vi "Set Output Operation State.vi"(0 "VISA resource name":refnum<visa-resource-name>, 1 "Voltage Setpoint (0 V)":dbl format="%#.6g", 2 "Current Setpoint (0 A)":dbl format="%#.6g", 5 "Mode (0: Off)":i32(ring) items=["Off", "Standby", "Charge", "Discharge", "Battery"], 7 "Enable":T1, 11 "error in (no error)":errorcluster, 12 "Power Setpoint (0 W)":dbl format="%#.6g", 13 "Resistance Setpoint (0 Ohms)":dbl format="%#.6g") -> (4 "VISA resource name out":refnum<visa-resource-name>, 15 "error out":errorcluster)   [LabVIEW 2020, in "NH Research Regenerative Test Series.lvlib"]
doc: "This command sets the operation mode and settings."
uses:
  Drivers-Essentials/NH Research Regenerative Test Series.lvlib
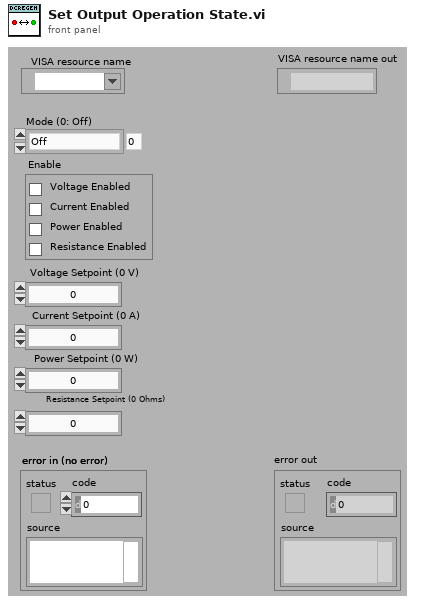
[diagram p1: front panel]
types:
  T1 = cluster{"Voltage Enabled":bool, "Current Enabled":bool, "Power Enabled":bool, "Resistance Enabled":bool}
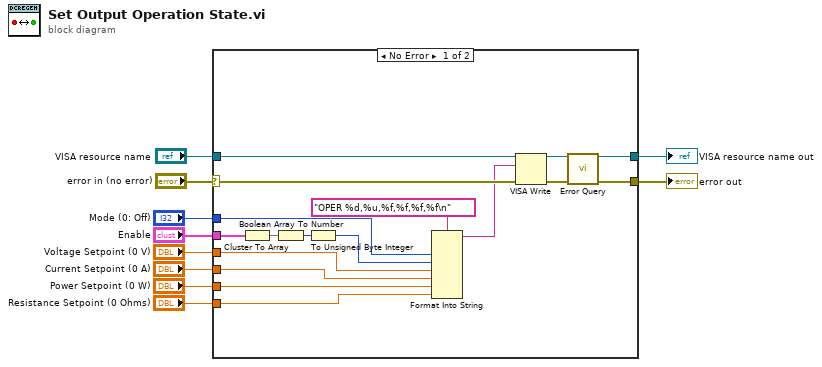
[diagram p0: block diagram]
diagram:
  n1 = case shown="No Error" "error in (no error)" {
    selector: "error in (no error)" -> [w22 w29]
    tunnel: "VISA resource name" -> [w27 w28]
    tunnel: [w26 w28] -> w9
    tunnel: [w25 w29] -> w8
    tunnel: "Enable" -> [w18 _]
    tunnel: "Mode (0: Off)" -> [w15 _]
    tunnel: "Voltage Setpoint (0 V)" -> [w14 _]
    tunnel: "Current Setpoint (0 A)" -> [w13 _]
    tunnel: "Power Setpoint (0 W)" -> [w12 _]
    tunnel: "Resistance Setpoint (0 Ohms)" -> [w11 _]
    frame No Error {
      n2 = Cluster To Array(cluster=w18) -> (array=w17:bool[])
      n3 = Boolean Array To Number(Boolean array=w17) -> (number=w19:u32)
      n4 = To Unsigned Byte Integer(number=w19) -> (unsigned 8bit integer=w16:u8)
      n5 = Format Into String(format string="OPER %d,%u,%f,%f,%f,%f\n", w15, w16, w14, w13, w12, w11) -> (resulting string=w20:string)  [unwired: 2 in, 1 out]
      n6 = VISA Write(VISA resource name=w27, write buffer=w20, error in (no error)=w22) -> (VISA resource name out=w24:refnum<visa-resource-name>, error out=w23:errorcluster)  [unwired: 1 out]
      n7 = call "Error Query.vi"("VISA resource name"=w24, "error in (no error)"=w23) -> ("VISA resource name out"=w26:refnum<visa-resource-name>, "error out"=w25:errorcluster)  [unwired: 10 in, 2 out]
    }
    frame Error {
    }
  }
  "error out" <- w8
  "VISA resource name out" <- w9
